vi "Switch Open Refs.vi"(8 "error in (no error)":errorcluster, 11 "JSONCluster":T1) -> (0 "error out":errorcluster, 3 "Switch Refs":refnum<k15>[](array[refnum]))   [LabVIEW 2019]
uses:
  JSONCluster.ctl
  <instrlib>/niSwitch/niSwitch.llb/niSwitch Topologies.ctl
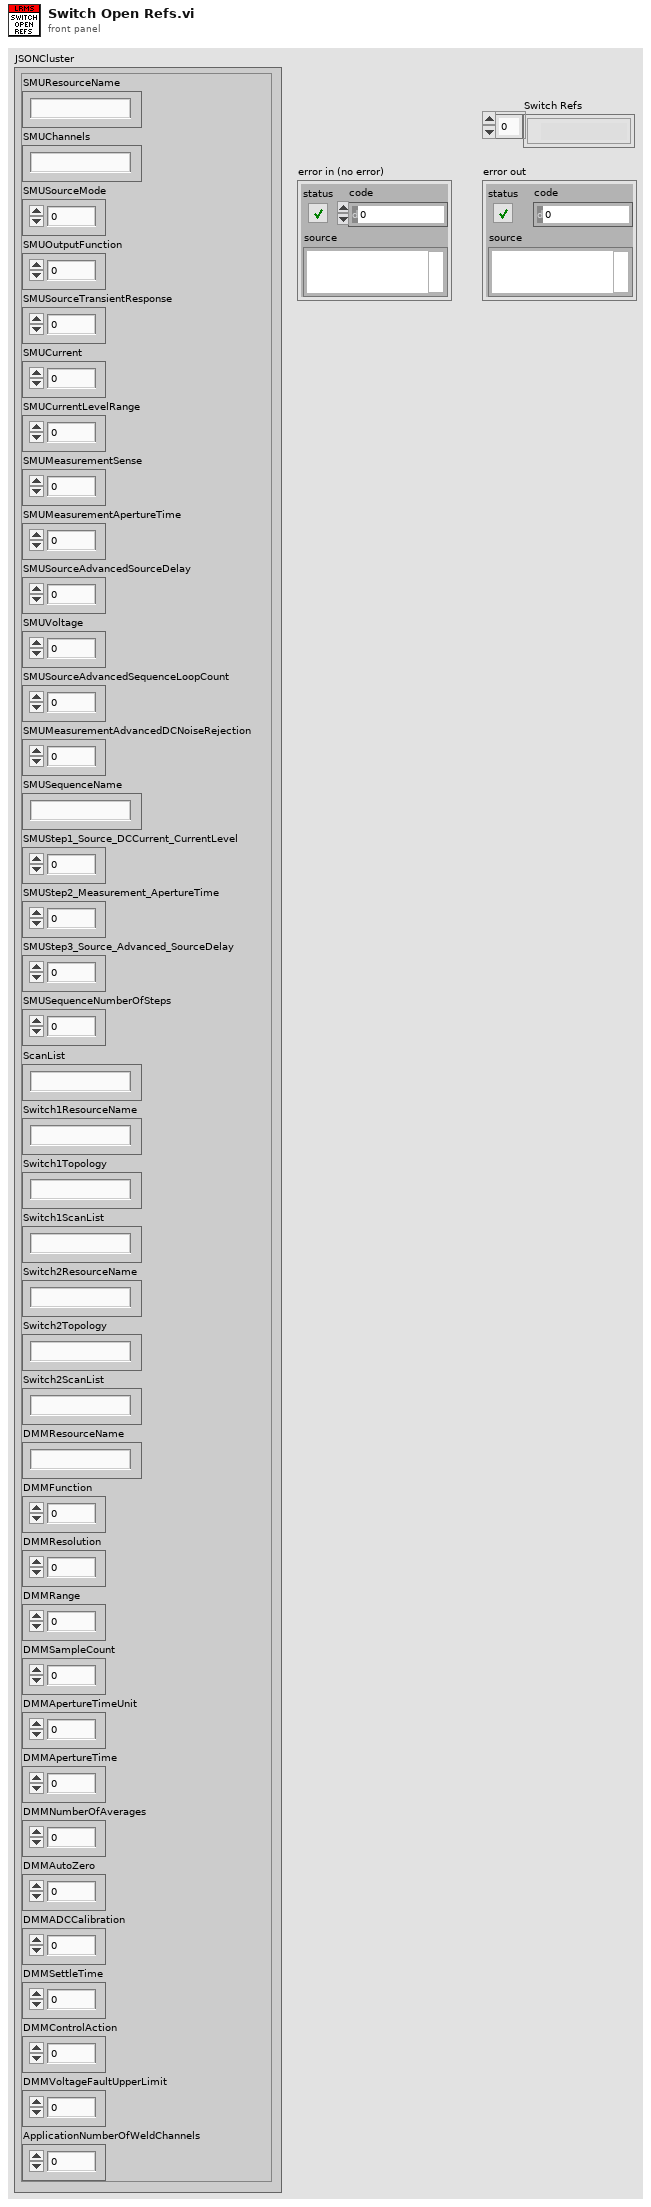
[diagram p1: front panel]
types:
  T1 = typedef "JSONCluster.ctl" = cluster{"SMUResourceName":string, "SMUChannels":string, "SMUSourceMode":i32, "SMUOutputFunction":i32, "SMUSourceTransientResponse":i32, "SMUCurrent":dbl, "SMUCurrentLevelRange":dbl, "SMUMeasurementSense":i32, "SMUMeasurementApertureTime":dbl, "SMUSourceAdvancedSourceDelay":dbl, "SMUVoltage":dbl, "SMUSourceAdvancedSequenceLoopCount":i32, "SMUMeasurementAdvancedDCNoiseRejection":i32, "SMUSequenceName":string, "SMUStep1_Source_DCCurrent_CurrentLevel":i32, "SMUStep2_Measurement_ApertureTime":i32, "SMUStep3_Source_Advanced_SourceDelay":i32, "SMUSequenceNumberOfSteps":i32, "ScanList":string, "Switch1ResourceName":string, "Switch1Topology":string, "Switch1ScanList":string, "Switch2ResourceName":string, "Switch2Topology":string, "Switch2ScanList":string, "DMMResourceName":string, "DMMFunction":i32, "DMMResolution":dbl, "DMMRange":dbl, "DMMSampleCount":i32, "DMMApertureTimeUnit":i32, "DMMApertureTime":dbl, "DMMNumberOfAverages":i32, "DMMAutoZero":i32, "DMMADCCalibration":i32, "DMMSettleTime":dbl, "DMMControlAction":i32, "DMMVoltageFaultUpperLimit":dbl, "ApplicationNumberOfWeldChannels":i32}
  T2 = typedef "niSwitch Topologies.ctl" = string
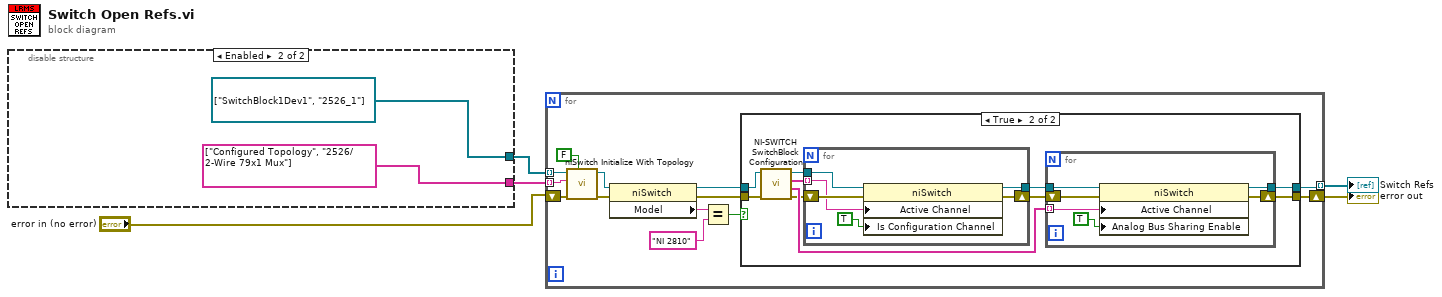
[diagram p0: block diagram]
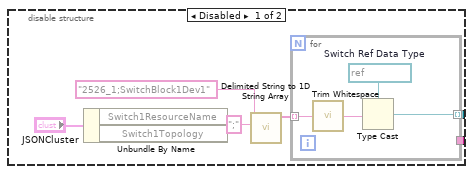
[diagram p2: hidden frame]
diagram:
  n1 = disable-structure shown="Enabled" {
    disable-tunnel: [w7 refnum<k15>[] ["SwitchBlock1Dev1", "2526_1"]] -> w2
    disable-tunnel: [_ T2[] ["Configured Topology", "2526/2-Wire 79x1 Mux"]] -> w1
    frame Disabled {
      n2 = Unbundle By Name("JSONCluster") -> ()  [unwired: 2 out]
      n3 = call <vilib>:"Delimited String to 1D String Array.vi"("delimiter"=";", "delimited string"="2526_1;SwitchBlock1Dev1") -> ("string array"=w8:string[])  [unwired: 9 in]
      n4 = for {
        tunnel: w8 -> [w14] mode=indexing
        tunnel: [w11] -> w7 mode=indexing
        w13 = refnum<k15> "2526_1"  # Switch Ref Data Type
        n5 = call <vilib>:"Trim Whitespace.vi"("string"=w14) -> ("trimmed string"=w12:string)  [unwired: 1 in]
        n6 = Type Cast(type=w13, x=w12) -> (*(type *) &x=w11:refnum<k15>)
      }
    }
    frame Enabled {
    }
  }
  n7 = for {
    tunnel: w2 -> [w29] mode=indexing
    shift-right: [w19] -> w4
    shift-left: "error in (no error)" -> [w27]
    tunnel: [w18] -> w3 mode=indexing
    tunnel: w1 -> [w17] mode=indexing
    n8 = call <instrlib>:"niSwitch Initialize With Topology.vi"("simulate (boolean value)"=FALSE, "error in (no error)"=w27, "topology name"=w17, "resource name"=w29) -> ("error out"=w25:errorcluster, "instrument handle out"=w26:refnum<k15>)  [unwired: 6 in]
    n9 = property class="niSwitch"(reference=w26, error in=w25) -> (reference out=w23:refnum<k15>, error out=w24:errorcluster, "Model"=w22:string)
    n10 = Equal?(x=w22, y="NI 2810") -> (x = y?=w20:bool)
    n11 = case shown="True" w20 {
      tunnel: [w31 w38] -> w18
      tunnel: [w30 w37] -> w19
      tunnel: w24 -> [w30 w35]
      tunnel: w23 -> [w31 w34]
      frame False {
      }
      frame True {
        n12 = call "NI-SWITCH SwitchBlock Configuration.vi"("error in (no error)"=w35, "Reference In"=w34) -> ("error out"=w32:errorcluster, "Analog Bus Array"=w33:string[], "Row Array"=w40:string[], "Reference out"=w36:refnum<k15>)  [unwired: 6 in]
        n13 = for {
          tunnel: w40 -> [w50] mode=indexing
          shift-right: [w52] -> w39
          shift-left: w32 -> [w51]
          tunnel: w36 -> [w49]
          tunnel: [w48] -> w41
          n14 = property class="niSwitch"(reference=w49, error in=w51, "Active Channel"=w50, "Is Configuration Channel"=TRUE ("Channel Configuration:Is Configuration Channel")) -> (reference out=w48:refnum<k15>, error out=w52:errorcluster)
        }
        n15 = for {
          shift-right: [w44] -> w37
          shift-left: w39 -> [w45]
          tunnel: w41 -> [w46]
          tunnel: [w43] -> w38
          tunnel: w33 -> [w42] mode=indexing
          n16 = property class="niSwitch"(reference=w46, error in=w45, "Active Channel"=w42, "Analog Bus Sharing Enable"=TRUE ("Channel Configuration:Is Configuration Channel")) -> (reference out=w43:refnum<k15>, error out=w44:errorcluster)
        }
      }
    }
  }
  "Switch Refs" <- w3
  "error out" <- w4
